vi "AVI Video Conditional Close.vi"(8 "error in (no error)":errorcluster, 11 "Logging queue element in":T1={"Imaging Protocol"=enum."Live Imaging", "Number of Trials"=0, "Frame Size"=512, "# Averaged frames"=0, "Dwell time (us)"=0.0, "Index of Z-plane"=0, "Timelapse?"=FALSE, "Logging process is active"=FALSE, "Speed logging enabled"=FALSE, "tdms file ref"=refnum, "path"=path "", "Trial Number"=0, "Expected # points acquired"=FALSE, "Manually stopped"=FALSE, "Last trial"=FALSE, "Ch0 data"=[], "Ch1 data"=[], "Image Time"=[], "Continuous Time"=[], "Points acquired"={"Ch0 last trial"=0, "Ch1 last trial"=0, "All trials"=0}, "HW Timings File"=refnum} {"Frame Size" items=["100X100"=100, "128X128"=128, "200X200"=200, "256X256"=256, "512X512"=512, "1024x1024"=1024, "2048x2048"=2048]; "Dwell time (us)" format="%#.6g"}) -> (0 "error out":errorcluster)   [LabVIEW 2017]
uses:
  Typedefs/Logging queue element.ctl
  Typedefs/Imaging Protocols enum.ctl
  Typedefs/Frame Size.ctl
  Typedefs/Acquired points count.ctl
  Globals/gl_Binary time series files globals.vi
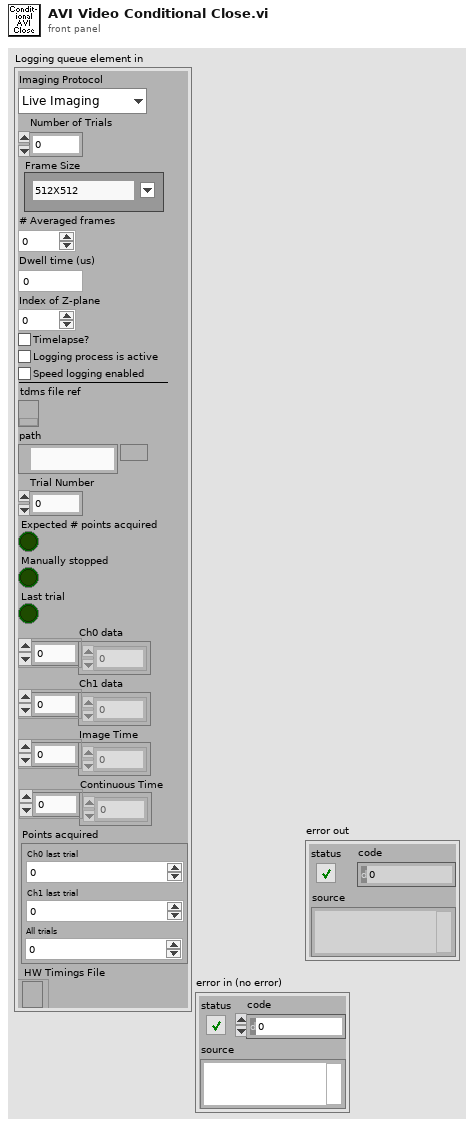
[diagram p1: front panel]
types:
  T1 = typedef "Logging queue element.ctl" = cluster{"Imaging Protocol":T2, "Number of Trials":u16, "Frame Size":T3, "# Averaged frames":u16, "Dwell time (us)":dbl, "Index of Z-plane":i32, "Timelapse?":bool, "Logging process is active":bool, "Speed logging enabled":bool, "tdms file ref":refnum<k34>, "path":path, "Trial Number":i32, "Expected # points acquired":bool, "Manually stopped":bool, "Last trial":bool, "Ch0 data":u32[], "Ch1 data":u32[], "Image Time":u64[], "Continuous Time":u64[], "Points acquired":T4, "HW Timings File":refnum<file>}
  T2 = typedef "Imaging Protocols enum.ctl" = enum16{"AOL Z-Stack", "Motor Z Stack", "Functional Acquisition", "Single Plane Acquisition", "Volume Acquisition", "Live Imaging", "Live Plane Imaging", "Live Volume Imaging"}
  T3 = typedef "Frame Size.ctl" = u16
  T4 = typedef "Acquired points count.ctl" = cluster{"Ch0 last trial":u64, "Ch1 last trial":u64, "All trials":u64}
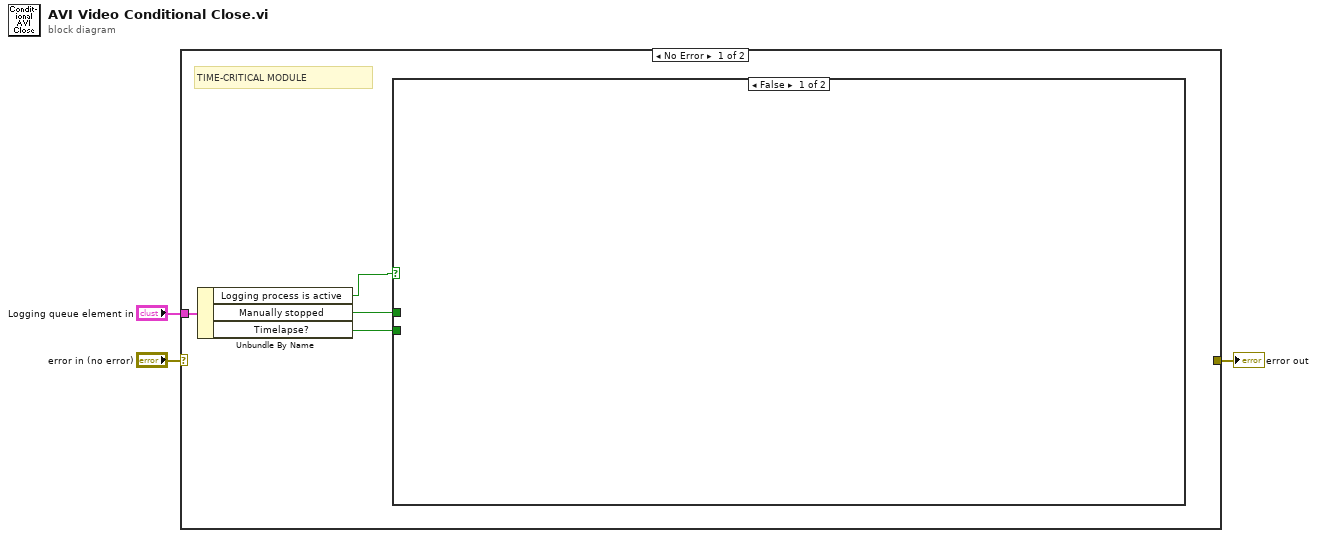
[diagram p0: block diagram]
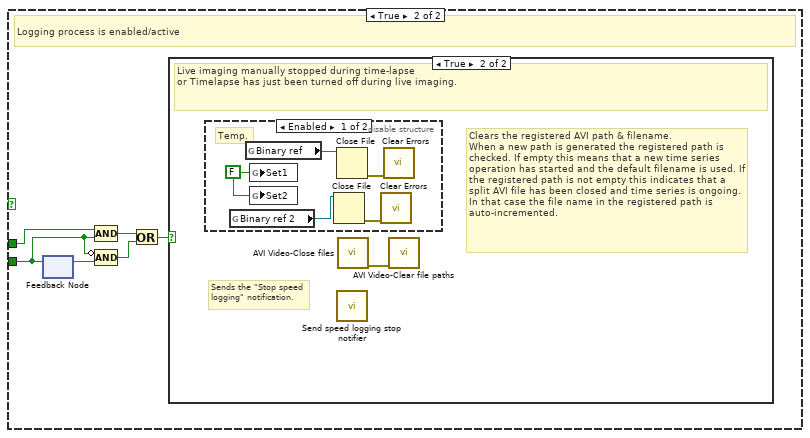
[diagram p2: hidden frame]
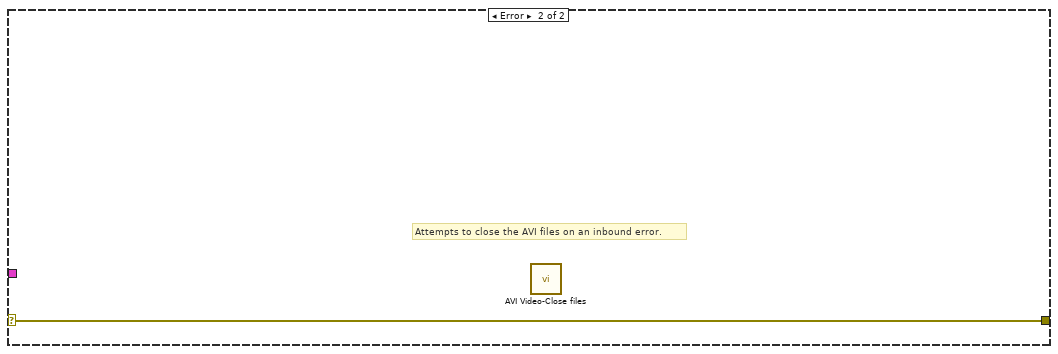
[diagram p5: hidden frame]
diagram:
  n1 = case shown="No Error" "error in (no error)" {
    selector: "error in (no error)" -> [_ w20]
    tunnel: "Logging queue element in" -> [w7 _]
    tunnel: [_ w20] -> w1
    frame No Error {
      # "TIME-CRITICAL MODULE"
      n2 = Unbundle By Name(w7) -> ("Logging process is active"=w4:bool, "Manually stopped"=w5:bool, "Timelapse?"=w6:bool)
      n3 = case shown="False" w4 {
        tunnel: w6 -> [_ w10]
        tunnel: w5 -> [_ w9]
        frame False {
        }
        frame True {
          # "Logging process is enabled/active"
          n4 = feedback #1() -> (w12:bool)  [unwired: 1 in]
          n5 = feedback-in #1(w10) -> ()
          n6 = Compound Arithmetic op=AND(w9, w10) -> (w8:bool)
          n7 = Compound Arithmetic op=AND(invert w10, w12) -> (w11:bool)
          n8 = Or(x=w8, y=w11) -> (x .or. y?=w13:bool)
          n9 = case shown="True" w13 {
            frame False {
              # "Not stopped"
            }
            frame True {
              # "Sends the \"Stop speed logging\" notification."
              # "Clears the registered AVI path & filename.\nWhen a new path is generated the registered path is checked. If empty this means that a new time series operation has started and the default filename is used. If the registered path is not empty this indicates that a split AVI file has been closed and time series is ongoing. In that case the file name in the registered path is auto-incremented."
              # "Live imaging manually stopped during time-lapse\nor Timelapse has just been turned off during live imaging."
              n10 = disable-structure shown="Enabled" {
                frame Enabled {
                  w15 = FALSE ("Set1")
                  # "Temp."
                  n11 = global read "gl_Binary time series files globals.vi" "Binary ref 2"() -> (w16:refnum<file>)
                  n12 = global read "gl_Binary time series files globals.vi" "Binary ref"() -> (w19:refnum<file>)
                  n13 = global write "gl_Binary time series files globals.vi" "Set1"(w15) -> ()
                  n14 = global write "gl_Binary time series files globals.vi" "Set2"(w15) -> ()
                  n15 = Close File(refnum=w16) -> (error out=w17:errorcluster)  [unwired: 1 in, 1 out]
                  n16 = Close File(refnum=w19) -> (error out=w18:errorcluster)  [unwired: 1 in, 1 out]
                  n17 = call <vilib>:"Clear Errors.vi"("error in (no error)"=w17) -> ()  [unwired: 5 in, 2 out]
                  n18 = call <vilib>:"Clear Errors.vi"("error in (no error)"=w18) -> ()  [unwired: 5 in, 2 out]
                }
                frame Disabled {
                }
              }
              n19 = call "Send speed logging stop notifier.vi"() -> ()  [unwired: 11 in, 1 out]
              n20 = call "AVI Video-Close files.vi"() -> ("error out (pass through)"=w14:errorcluster)  [unwired: 11 in]
              n21 = call "AVI Video-Clear file paths.vi"("error in (no error)"=w14) -> ()  [unwired: 10 in, 1 out]
            }
          }
        }
      }
    }
    frame Error {
      # "Attempts to close the AVI files on an inbound error."
      n22 = call "AVI Video-Close files.vi"() -> ()  [unwired: 11 in, 1 out]
    }
  }
  "error out" <- w1
